vi "Publisher.vi"() -> ()   [LabVIEW 2020]
uses:
  Global 1.vi
panel:
  in  "stop":bool
  in  "Publisher":dbl
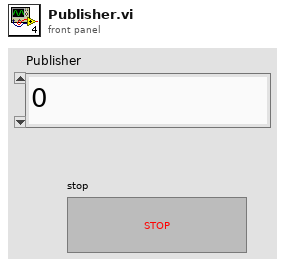
[diagram p1: front panel]
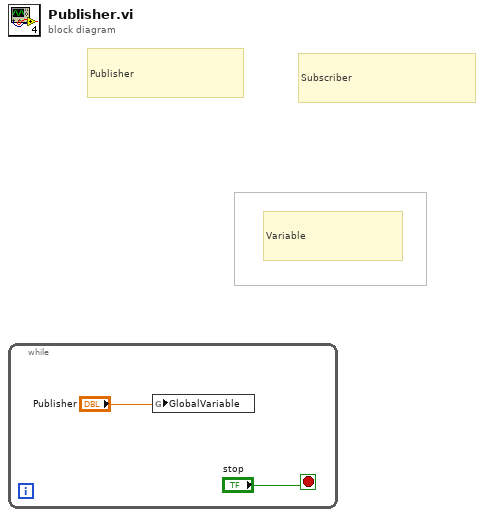
[diagram p0: block diagram]
diagram:
  # "Variable"
  # "Subscriber"
  # "Publisher"
  n1 = while {
    stop <- "stop" stop-if-true
    n2 = global write "Global 1.vi" "GlobalVariable"("Publisher") -> ()
  }
